vi "Verify as JSON.vi"(5 "Label":string, 7 "Approval Tests.lvlib:Options.lvclass":refnum<class "Options.lvclass">, 8 "error in":errorcluster, 10 "Anything":variant) -> (0 "error out":errorcluster, 1 "Failure Message":string, 2 "Passed?":bool)   [LabVIEW 2020, in "Approval Tests.lvlib"]
doc: "Takes in anything. Flattens it to JSON."
uses:
  Approval Tests.lvlib
  Text Comparator/Text Comparator.lvclass
  JSON Comparator/JSON Comparator.lvclass
  446ea483-69c6-4b80-9828-6e8c6966e28d.vi
  <vilib>/PNR/JSONtext Object Serialization/Generic Object Serializer/Generic Object Serializer.lvclass
  Options/Options.lvclass
  Naming Data/Naming Data.lvclass
  80a56ea5-82bd-4847-ab10-a71bf4fcdb91.vi
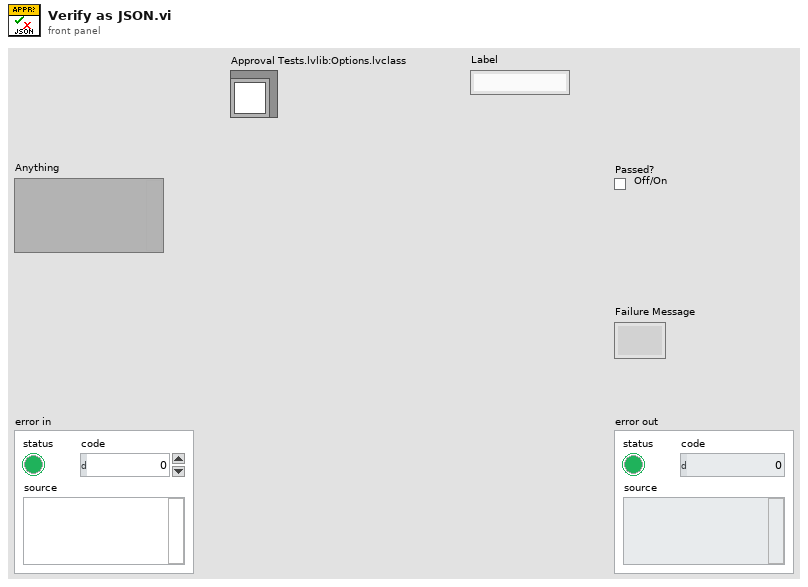
[diagram p1: front panel]
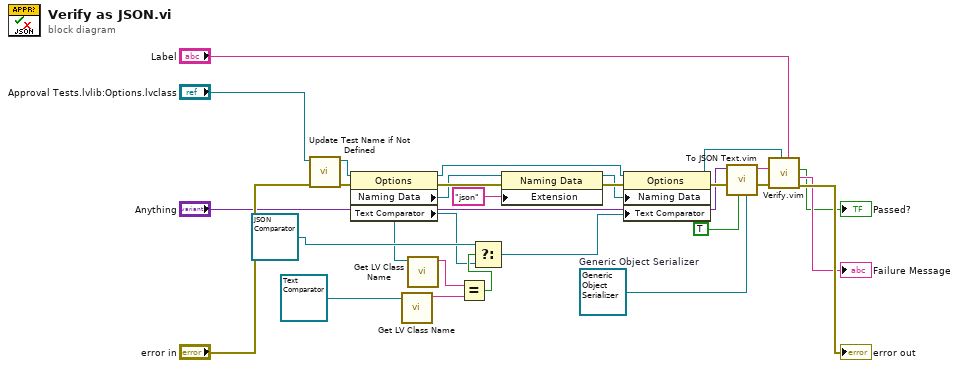
[diagram p0: block diagram]
diagram:
  w17 = refnum<class "Generic Object Serializer.lvclass"> refnum  # Generic Object Serializer
  n1 = call "Update Test Name if Not Defined.vi"("error in"="error in", "Options in"="Approval Tests.lvlib:Options.lvclass") -> ("error out"=w25:errorcluster, "Options out"=w10:refnum<class "Options.lvclass">)  [unwired: 8 in]
  n2 = property class="Options"(reference=w10, error in=w25) -> (reference out=w15:refnum<class "Options.lvclass">, error out=w24:errorcluster, "Naming Data"=w14:refnum<class "Naming Data.lvclass">, "Text Comparator"=w3:refnum<class "Text Comparator.lvclass">)
  n3 = call <vilib>:"Get LV Class Name.vi"("object"=refnum<class "Text Comparator.lvclass"> refnum ("Approval Tests:Text Comparator")) -> ("class name"=w5:string)  [unwired: 9 in, 1 out]
  n4 = call <vilib>:"Get LV Class Name.vi"("object"=w3) -> ("class name"=w6:string)  [unwired: 9 in, 1 out]
  n5 = Equal?(x=w6, y=w5) -> (x = y?=w4:bool)
  n6 = Select(t=refnum<class "JSON Comparator.lvclass"> refnum ("Approval Tests:JSON Comparator.lvclass"), s=w4, f=w3) -> (s? t:f=w2:refnum<class "Text Comparator.lvclass">)
  n7 = property class="Naming Data"(reference=w14, error in=w24, "Extension"="json" ("Extension(txt)")) -> (reference out=w13:refnum<class "Naming Data.lvclass">, error out=w23:errorcluster)
  n8 = property class="Options"(reference=w15, error in=w23, "Naming Data"=w13, "Text Comparator"=w2) -> (reference out=w1:refnum<class "Options.lvclass">, error out=w22:errorcluster)
  n9 = call "To JSON Text.vim"("LVClass Serializer"=w17, "Pretty Print?"=TRUE, "error in (no error)"=w22, "Anything"="Anything") -> ("error out"=w26:errorcluster, "<JSON>"=w18:string)  [unwired: 6 in]
  n10 = call "Verify.vim"("Label"="Label", "Options"=w1, "error in"=w26, "Anything"=w18) -> ("error out"=→"error out":errorcluster, "Failure Message"=→"Failure Message":string, "Passed?"=→"Passed?":bool)  [unwired: 5 in]
